vi "Get status.vi"(8 "error in (no error)":errorcluster, 11 "RT Management in":refnum<class "RT Management.lvclass">) -> (0 "error out":errorcluster, 1 "Status string":string, 2 "Status":T1, 3 "RT Management out":refnum<class "RT Management.lvclass">)   [LabVIEW 2015, in "RT Management.lvlib" / "RT Management.lvclass"]
doc: "This VI returns the status of the RT target. This method relies on the System Configuration API's Real-Time:System Status property, which is returned as a string. In the case that a new status string is added that isn't accounted for by this VI, the value \"Unknown\" will be returned. You can then check the \"Status string\" indicator for what was returned by the System Configuration API.\n\nSome common values: Unknown, Disconnected, Running, Unconfigured, Install Mode, No software installed, Safe Mode (User Directed), Safe Mode (No Software Installed)"
uses:
  RT Management.lvclass
  Controls/Status.ctl
  RT Management.lvclass/RT Management.ctl
  Get SysCfg Session.vi
  <resource>/objmgr/nisysapi.rc
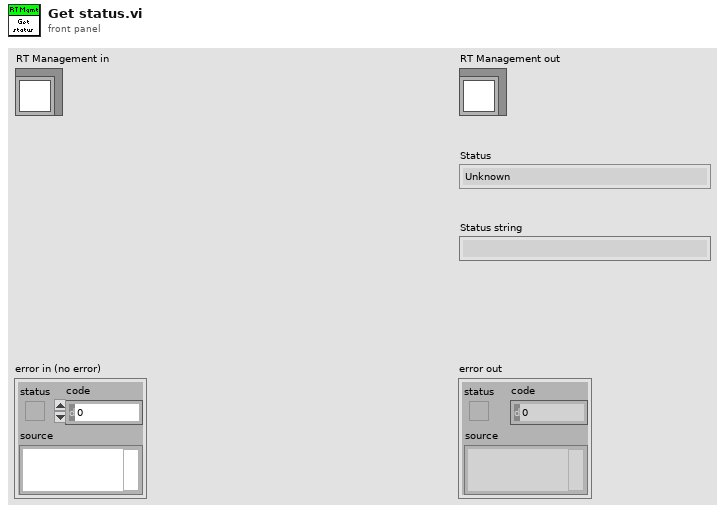
[diagram p1: front panel]
types:
  T1 = typedef "RT Management.lvlib/RT Management.lvclass/Status.ctl" = enum16{"Unknown", "Disconnected", "Running", "Unconfigured", "Install Mode", "No software installed", "Safe Mode (Corrupt Main Exe)", "Safe Mode (User Directed)", "Safe Mode (User Directed - Forced)", "Safe Mode (Software Error)", "Safe Mode (No Software Installed)", "Safe Mode (Corrupt Installation)", "Safe Mode (Improper Installation)", "Safe Mode (Main Program Not Found)", "Safe Mode (Software Update Required)", "Safe Mode (Unsupported RT Boot Partition)"}
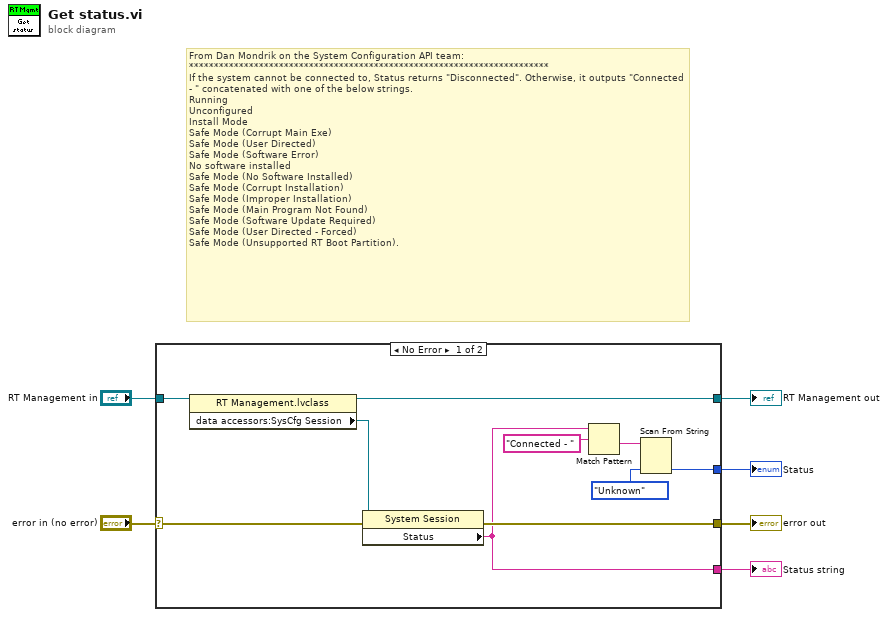
[diagram p0: block diagram]
diagram:
  # "From Dan Mondrik on the System Configuration API team:\n************************************************************************\nIf the system cannot be connected to, Status returns \"Disconnected\". Otherwise, it outputs \"Connected - \" concatenated with one of the below strings.\nRunning  \nUnconfigured \nInstall Mode\nSafe Mode (Corrupt Main Exe)\nSafe Mode (User Directed) \nSafe Mode (Software Error)\nNo software installed\nSafe Mode (No Software Installed)\nSafe Mode (Corrupt Installation) \nSafe Mode (Improper Installation)\nSafe Mode (Main Program Not Found)  \nSafe Mode (Software Update Required) \nSafe Mode (User Directed - Forced)  \nSafe Mode (Unsupported RT Boot Partition)."
  n1 = case shown="No Error" "error in (no error)" {
    selector: "error in (no error)" -> [w12 w18]
    tunnel: [w16 w18] -> w5
    tunnel: [w14 w17] -> w3
    tunnel: "RT Management in" -> [w15 w17]
    tunnel: [w10 _] -> w2
    tunnel: [w7 _] -> w1
    frame No Error {
      n2 = property class="RT Management.lvclass"(reference=w15) -> (reference out=w14:refnum<class "RT Management.lvclass">, "data accessors:SysCfg Session"=w13:refnum<k21>)  [unwired: 1 in, 1 out]
      n3 = property class="System Session"(reference=w13, error in=w12) -> (error out=w16:errorcluster, "Status"=w7:string)  [unwired: 1 out]
      n4 = Match Pattern(string=w7, regular expression="Connected - ") -> (after substring=w8:string)  [unwired: 1 in, 3 out]
      n5 = Scan From String(input string=w8, default 1=Status."Unknown" ("Status")) -> (output 1=w10:T1)  [unwired: 3 in, 3 out]
    }
    frame Error {
    }
  }
  "error out" <- w5
  "RT Management out" <- w3
  "Status" <- w2
  "Status string" <- w1
